vi "Save Calibration.vi"(7 "Calibration Sensor":T2, 8 "error in (no error)":errorcluster, 11 "GlobalData":T1) -> (0 "error out":errorcluster)   [LabVIEW 2024]
doc: "Save Calibration Data into Config File"
uses:
  controls/Cal Sensor Enum.ctl
  controls/GlobalData.ctl
  <vilib>/Utility/config.llb/Write Key (String).vi
  <vilib>/Utility/config.llb/NI_LVConfig.lvlib
panel:
  out "success":bool
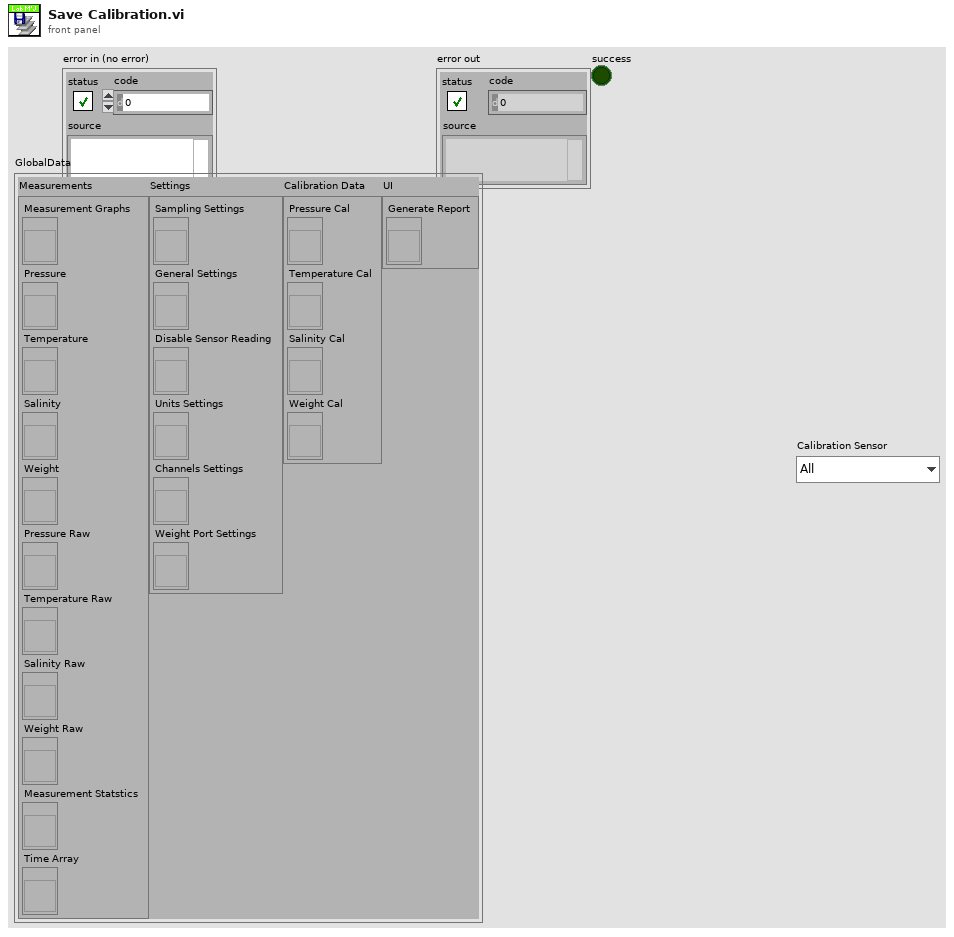
[diagram p1: front panel]
types:
  T1 = typedef "GlobalData.ctl" = cluster{"Measurements":cluster{"Measurement Graphs":refnum<vi>, "Pressure":refnum<vi>, "Temperature":refnum<vi>, "Salinity":refnum<vi>, "Weight":refnum<vi>, "Pressure Raw":refnum<vi>, "Temperature Raw":refnum<vi>, "Salinity Raw":refnum<vi>, "Weight Raw":refnum<vi>, "Measurement Statstics":refnum<vi>, "Time Array":refnum<vi>}, "Settings":cluster{"Sampling Settings":refnum<vi>, "General Settings":refnum<vi>, "Disable Sensor Reading":refnum<vi>, "Units Settings":refnum<vi>, "Channels Settings":refnum<vi>, "Weight Port Settings":refnum<vi>}, "Calibration Data":cluster{"Pressure Cal":refnum<vi>, "Temperature Cal":refnum<vi>, "Salinity Cal":refnum<vi>, "Weight Cal":refnum<vi>}, "UI":cluster{"Generate Report":refnum<vi>}}
  T2 = typedef "Cal Sensor Enum.ctl" = enum16{"All", "Pressure", "Temperature", "Salinity", "Weight"}
  T3 = cluster{"C (Y-Intercept)":dbl, "M (Gradient)":dbl}
  T4 = typedef "NI_LVConfig.lvlib/Config Data RefNum.ctl" = refnum<k1>
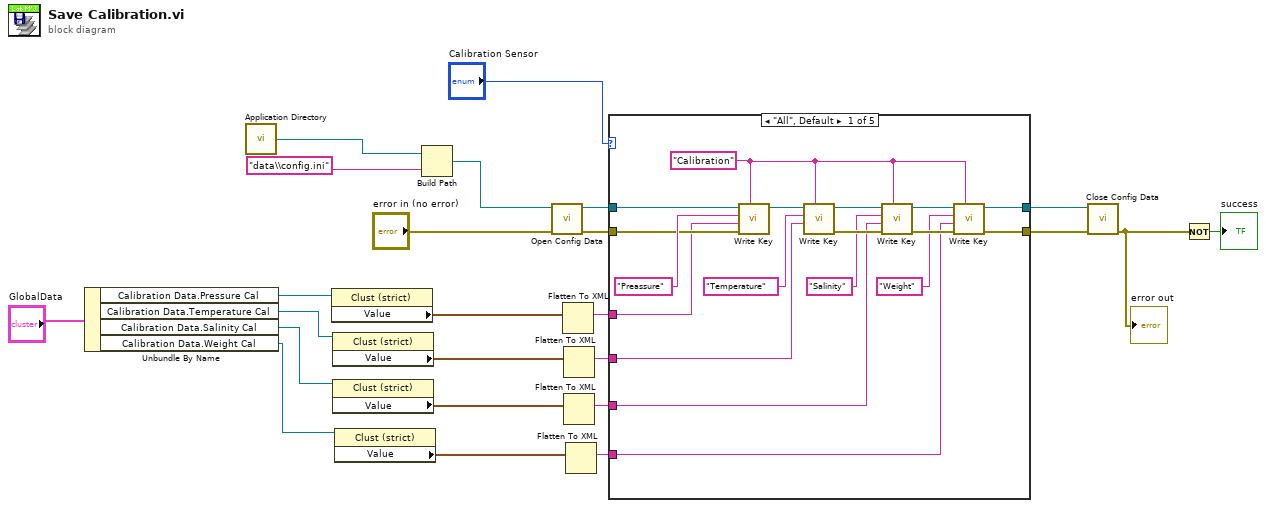
[diagram p0: block diagram]
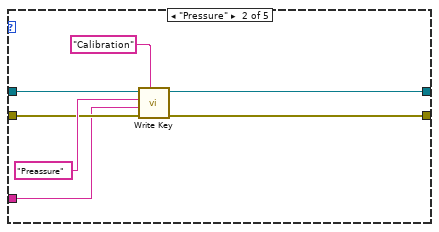
[diagram p2: hidden frame]
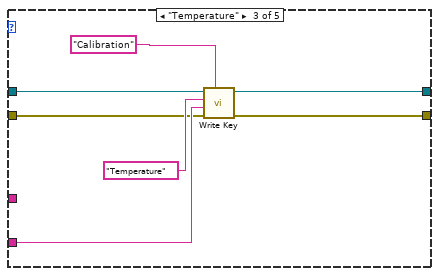
[diagram p3: hidden frame]
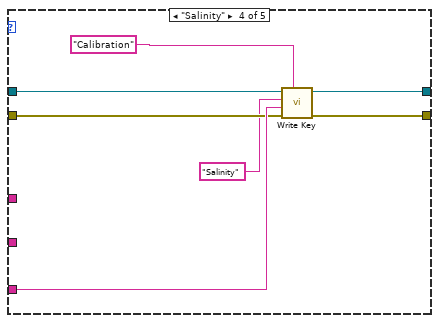
[diagram p4: hidden frame]
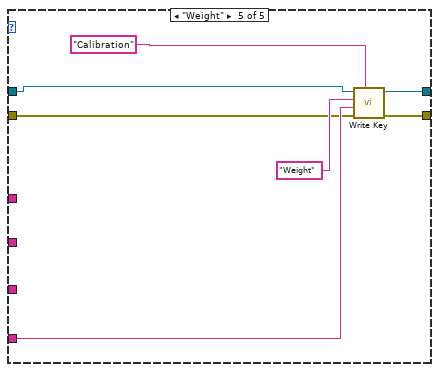
[diagram p5: hidden frame]
diagram:
  n1 = Unbundle By Name("GlobalData") -> ("Calibration Data.Pressure Cal"=w12:refnum<vi>, "Calibration Data.Temperature Cal"=w11:refnum<vi>, "Calibration Data.Salinity Cal"=w7:refnum<vi>, "Calibration Data.Weight Cal"=w8:refnum<vi>)
  n2 = call <vilib>:"Application Directory.vi"() -> ("Application Directory"=w15:path)
  n3 = property class="Clust (strict)"(reference=w12) -> ("Value"=w19:T3)  [unwired: 1 in, 2 out]
  n4 = property class="Clust (strict)"(reference=w11) -> ("Value"=w17:T3)  [unwired: 1 in, 2 out]
  n5 = property class="Clust (strict)"(reference=w7) -> ("Value"=w10:T3)  [unwired: 1 in, 2 out]
  n6 = property class="Clust (strict)"(reference=w8) -> ("Value"=w9:T3)  [unwired: 1 in, 2 out]
  n7 = Build Path(base path=w15, name or relative path="data\\config.ini") -> (appended path=w13:path)
  n8 = call <vilib>:"Open Config Data.vi"("error in (no error)"="error in (no error)", "configuration file path"=w13) -> ("error out"=w23:errorcluster, "refnum"=w24:T4)  [unwired: 7 in, 1 out]
  n9 = Flatten To XML(6:w19) -> (2:w18:string)
  n10 = Flatten To XML(6:w17) -> (2:w16:string)
  n11 = Flatten To XML(6:w10) -> (2:w6:string)
  n12 = Flatten To XML(6:w9) -> (2:w5:string)
  n13 = case shown="\"All\", Default" "Calibration Sensor" {
    tunnel: w24 -> [w42 w49 w53 w59 w65]
    tunnel: w23 -> [w40 w47 w52 w58 w64]
    tunnel: w18 -> [w39 w46 _ _ _]
    tunnel: w16 -> [w36 _ w55 _ _]
    tunnel: w6 -> [w28 _ _ w62 _]
    tunnel: w5 -> [w27 _ _ _ w68]
    tunnel: [w26 w44 w50 w61 w67] -> w4
    tunnel: [w25 w43 w51 w60 w66] -> w3
    frame "All", Default {
      w31 = "Calibration" ("section")
      n14 = call-poly <vilib>:"Write Key.vi"("section"=w31, "error in (no error)"=w40, "value"=w39, "key"="Preassure", "refnum"=w42) -> ("refnum out"=w37:T4)  [unwired: 4 in, 2 out]
      n15 = call-poly <vilib>:"Write Key.vi"("section"=w31, "value"=w36, "key"="Temperature", "refnum"=w37) -> ("error out"=w34:errorcluster, "refnum out"=w35:T4)  [unwired: 5 in, 1 out]
      n16 = call-poly <vilib>:"Write Key.vi"("section"=w31, "error in (no error)"=w34, "value"=w28, "key"="Salinity", "refnum"=w35) -> ("error out"=w32:errorcluster, "refnum out"=w33:T4)  [unwired: 4 in, 1 out]
      n17 = call-poly <vilib>:"Write Key.vi"("section"=w31, "error in (no error)"=w32, "value"=w27, "key"="Weight", "refnum"=w33) -> ("error out"=w25:errorcluster, "refnum out"=w26:T4)  [unwired: 4 in, 1 out]
    }
    frame "Pressure" {
      n18 = call-poly <vilib>:"Write Key.vi"("section"="Calibration", "error in (no error)"=w47, "value"=w46, "key"="Preassure", "refnum"=w49) -> ("error out"=w43:errorcluster, "refnum out"=w44:T4)  [unwired: 4 in, 1 out]
    }
    frame "Temperature" {
      n19 = call-poly <vilib>:"Write Key.vi"("section"="Calibration", "error in (no error)"=w52, "value"=w55, "key"="Temperature", "refnum"=w53) -> ("error out"=w51:errorcluster, "refnum out"=w50:T4)  [unwired: 4 in, 1 out]
    }
    frame "Salinity" {
      n20 = call-poly <vilib>:"Write Key.vi"("section"="Calibration", "error in (no error)"=w58, "value"=w62, "key"="Salinity", "refnum"=w59) -> ("error out"=w60:errorcluster, "refnum out"=w61:T4)  [unwired: 4 in, 1 out]
    }
    frame "Weight" {
      n21 = call-poly <vilib>:"Write Key.vi"("section"="Calibration", "error in (no error)"=w64, "value"=w68, "key"="Weight", "refnum"=w65) -> ("error out"=w66:errorcluster, "refnum out"=w67:T4)  [unwired: 4 in, 1 out]
    }
  }
  n22 = call <vilib>:"Close Config Data.vi"("error in (no error)"=w3, "refnum"=w4) -> ("error out"=w21:errorcluster)  [unwired: 8 in, 1 out]
  "error out" <- w21
  n23 = Not(x=w21) -> (.not. x?=→"success":bool)
